vi "c_ctre_phoenix6_platform_has_schema.vi"(0 "Numeric":u8, 1 "String 2":string, 2 "Numeric 2":u16) -> (20 "String":string)   [LabVIEW 2025]
uses:
  <vilib>/Rock Robotics/WPI/ThirdParty/Phoenix-LabVIEW/Controls/DriverLib.ctl
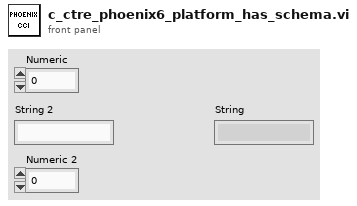
[diagram p1: front panel]
types:
  T1 = typedef "DriverLib.ctl" = path
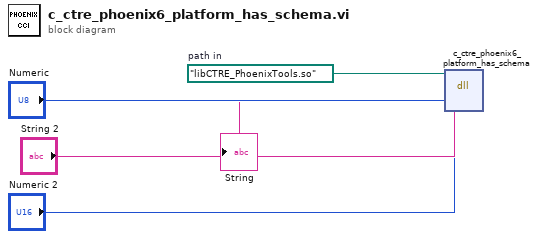
[diagram p0: block diagram]
diagram:
  w5 = T1 path "libCTRE_PhoenixTools.so"  # path in
  n1 = dll-call lib="?" fn="c_ctre_phoenix6_platform_has_schema"(path in=w5, "Numeric", "String 2", "Numeric 2") -> (→"String":string)  [unwired: 3 in, 2 out]
